vi "close_data_log.vi"(8 "error in (no error)":errorcluster, 11 "scan_hdf5_log in":refnum<class "scan_hdf5_log.lvclass">) -> (0 "error out":errorcluster, 3 "scan_hdf5_log out":refnum<class "scan_hdf5_log.lvclass">)   [LabVIEW 2015, in "scan_hdf5_log.lvclass"]
uses:
  scan_hdf5_log.lvclass
  scan_hdf5_log.lvclass/scan_hdf5_log.ctl
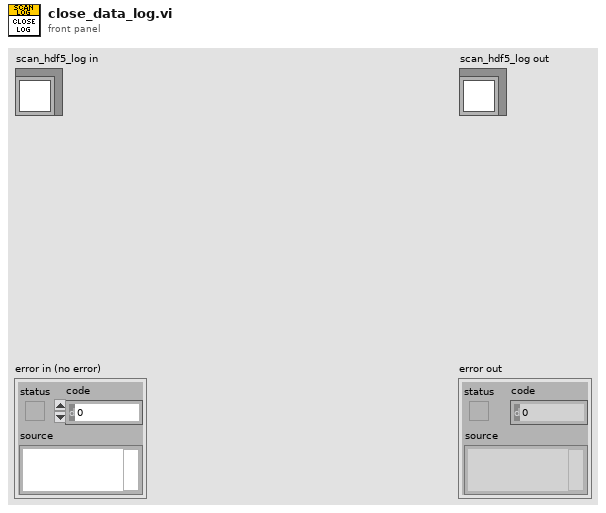
[diagram p1: front panel]
types:
  T1 = typedef "HDF5 Ref.ctl" = refnum<k1>
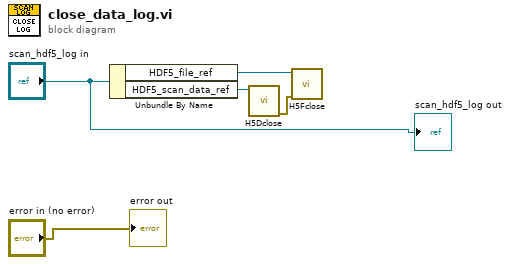
[diagram p0: block diagram]
diagram:
  n1 = Unbundle By Name("scan_hdf5_log in") -> ("HDF5_file_ref"=w5:T1, "HDF5_scan_data_ref"=w4:T1)
  n2 = call <vilib>:"H5Dclose.vi"("HDF5 Dataset Ref"=w4) -> ("error out"=w3:errorcluster)  [unwired: 8 in]
  n3 = call <vilib>:"H5Fclose.vi"("error in (no error)"=w3, "HDF5 Ref"=w5) -> ()  [unwired: 7 in, 1 out]
  "error out" <- "error in (no error)"
  "scan_hdf5_log out" <- "scan_hdf5_log in"
